vi "Real Matrix Norm.vi"(2 "norm type":T1 items=["2-norm", "1-norm", "F-norm", "Inf-norm"], 3 "Input Matrix":T2) -> (0 "error":i32, 1 "norm":dbl format="%.4f")   [LabVIEW 2017, in "NI_AALPro.lvlib"]
doc: "Computes the <B>norm</B> of <B>Input Matrix</B>. Wire data to the <B>Input Matrix</B> input to determine the polymorphic instance to use or manually select the instance."
uses:
  NI_AALPro.lvlib
  RealMatrix.ctl
  Matrix Norm Type.ctl
  <resource>/lvanlys.dll
  NI_Matrix.lvlib
panel:
  # "Matrix Norm"
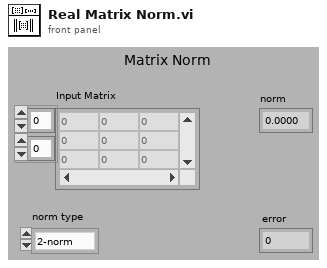
[diagram p1: front panel]
types:
  T1 = typedef "NI_AALPro.lvlib/Matrix Norm Type.ctl" = i32
  T2 = typedef "NI_Matrix.lvlib/RealMatrix.ctl" = dbl[][]
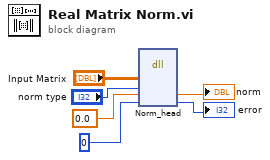
[diagram p0: block diagram]
diagram:
  n1 = dll-call lib="C:/Program Files (x86)/National Instruments/LabVIEW 2017/resource/lvanlys.*" fn="Norm_head"("Input Matrix"="Input Matrix", "norm type"="norm type", "output param"=0.0, "output param"=0) -> ("output param"=→"norm":dbl, "output param"=→"error":i32)  [unwired: 6 in, 2 out]
